vi "Main.vi"() -> ()   [LabVIEW 2025]
uses:
  Interlune UDP.ctl
  Enum_FileNewInterval.ctl
  <vilib>/DAQmx/read.llb/DAQmx Read (Analog 1D DBL NChan 1Samp).vi
  <vilib>/numeric/Random Number (Range) DBL.vi
  <extravilib>/ChannelInstances/Stream-a[.](dbl)/Read With Abort.vi
  <extravilib>/ChannelInstances/Stream-a[.](dbl)/Write With Abort.vi
  <extravilib>/ChannelInstances/Stream-a[.](dbl)/EndpointRead.vi
  <extravilib>/ChannelInstances/Stream-a[.](dbl)/Endpoint.vi
  <vilib>/DAQmx/miscellaneous.llb/DAQmx Fill In Error Info.vi
  <extravilib>/ChannelInstances/Stream-a[.](dbl)/Instantiate.vi
  <extravilib>/ChannelInstances/Stream-a[.](dbl)/)Channel.vi
  <resource>/ChannelSupport/_ChannelSupport/WaitIfNeeded.vi
  <extravilib>/ChannelInstances/Stream-a[.](dbl).lvlib
panel:
  in  "Output tabs":enum32{"Raw", "Cleaned"}(tab)
  out "LC Voltage Graph":T1(graph)
  out "Raw Voltages":dbl[](array[numeric])
  out "RAW UDP":string
  out "T Voltage Graph":cluster{"[0]":dbl}(graph)
  out "UDP Cluster":T2
  out "Forces":dbl[](array[numeric])
  out "LC Graph":T1(graph)
  out "T Graph":cluster{"[0]":dbl}(graph)
  in  "Load Cell Labeling":string[](array[string])=["LV1X", "LV1Y", "LV1Z", "LV2X", "LV2Y", "LV2Z", "LV3X", "LV3Y", "LV3Z", "LV4X", "LV4Y", "LV4Z"]
  in  "Torque Sensor":tag="cDAQ1Mod2/ai1"
  out "Time(s)":dbl
  in  "Emulation?":bool
  in  "Stop?":bool
  in  "Load Cells":tag[](array[tag])=["cDAQ1Mod1/ai5", "cDAQ1Mod1/ai4", "cDAQ1Mod1/ai6", "cDAQ1Mod1/ai8", "cDAQ1Mod1/ai7", "cDAQ1Mod1/ai9", "cDAQ1Mod1/ai11", "cDAQ1Mod1/ai10", "cDAQ1Mod1/ai12", "cDAQ1Mod1/ai14", "cDAQ1Mod1/ai13", "cDAQ1Mod1/ai15"]
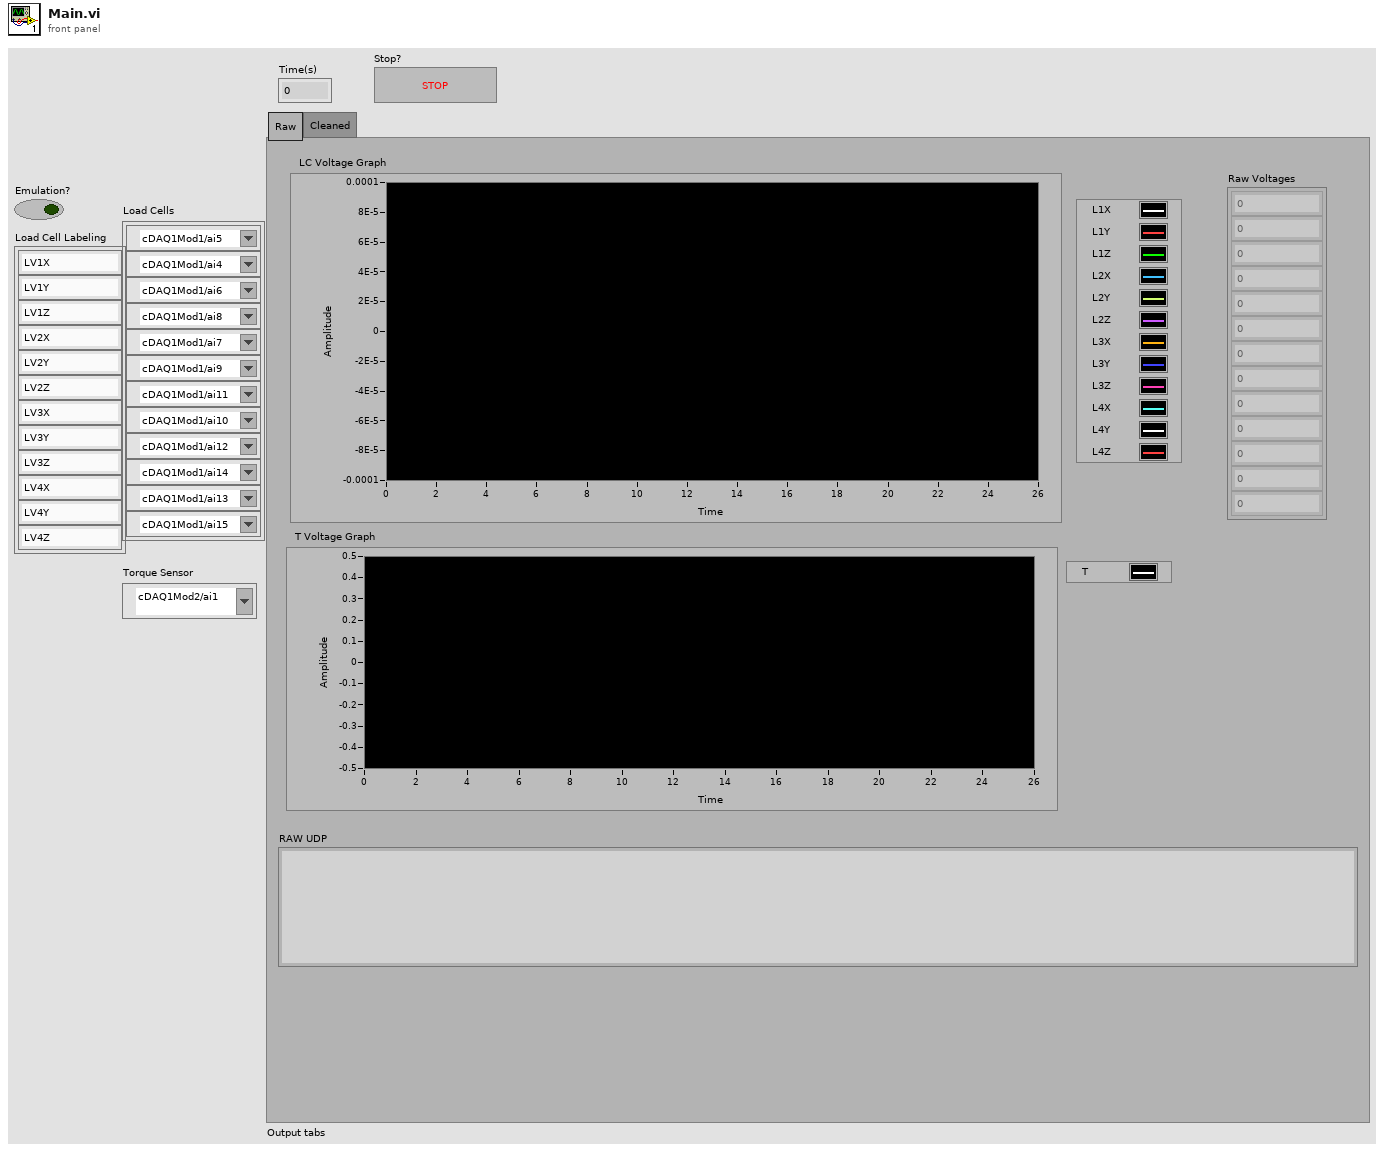
[diagram p1: front panel]
types:
  T1 = cluster{"[0]":dbl, "[1]":dbl, "[2]":dbl, "[3]":dbl, "[4]":dbl, "[5]":dbl, "[6]":dbl, "[7]":dbl, "[8]":dbl, "[9]":dbl, "[10]":dbl, "[11]":dbl}
  T2 = typedef "Interlune UDP.ctl" = cluster{"status":cluster{"ts_ms":dbl, "hw_estop":dbl, "motor_count":dbl}, "vertical":cluster{"has_v":dbl, "cmd":dbl, "raw_cmd":dbl, "velocity":dbl, "raw_velocity":dbl, "local_position":dbl, "global_position":dbl, "raw_position":dbl, "torque":dbl}, "horizontal":cluster{"has_h":dbl, "cmd":dbl, "raw_cmd":dbl, "velocity":dbl, "raw_velocity":dbl, "local_position":dbl, "global_position":dbl, "raw_position":dbl, "torque":dbl}, "attachment":cluster{"has_a":dbl, "cmd":dbl, "raw_cmd":dbl, "velocity":dbl, "raw_velocity":dbl, "global_position":dbl, "raw_position":dbl, "torque":dbl}}
  T3 = enum16{"open", "open or create", "create or replace", "create", "open (read-only)"}
  T4 = typedef "Enum_FileNewInterval.ctl" = enum16{"2 Min", "10 Min", "Hourly", "Daily", "Weekly", "Monthly"}
  T5 = typedef "Stream-a[.](dbl).lvlib/)Channel.ctl" = refnum<queue>
  T6 = cluster{"[0]":dbl, "[1]":dbl, "[2]":dbl, "[3]":dbl, "[4]":dbl, "[5]":dbl, "[6]":dbl, "[7]":dbl, "[8]":dbl, "[9]":dbl, "[10]":dbl, "[11]":dbl, "[12]":dbl}
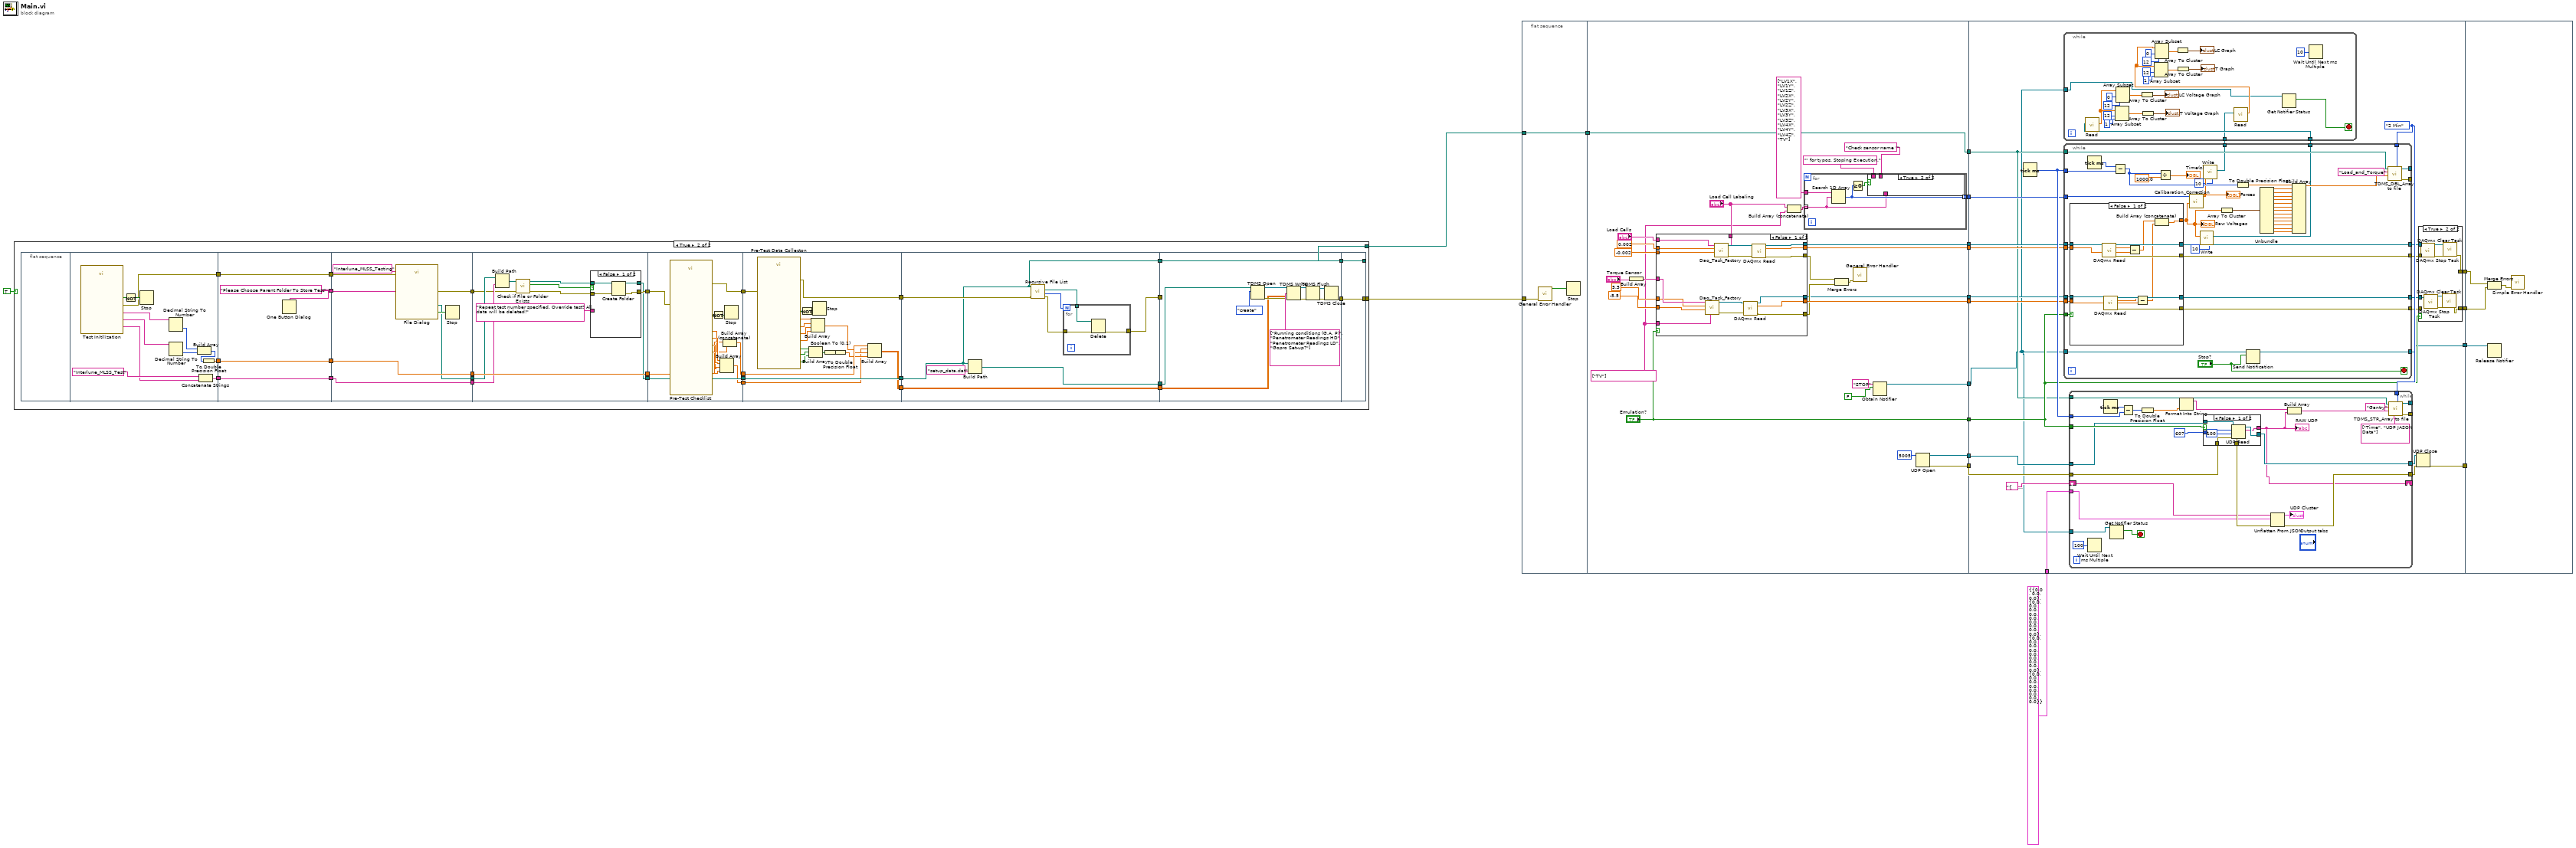
[diagram p0: block diagram]
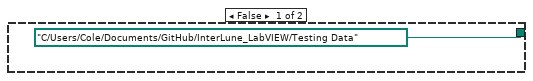
[diagram p2: hidden frame]
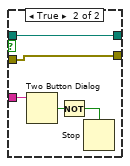
[diagram p3: hidden frame]
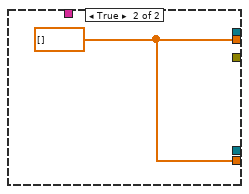
[diagram p4: hidden frame]
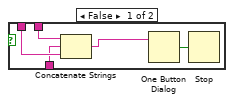
[diagram p5: hidden frame]
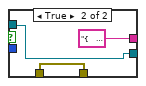
[diagram p7: hidden frame]
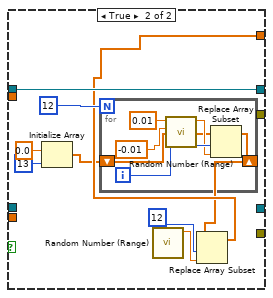
[diagram p8: hidden frame]
diagram:
  n1 = case shown="True" TRUE {
    tunnel: [_ w29] -> w12
    tunnel: [path "C:/Users/Cole/Documents/GitHub/InterLune_LabVIEW/Testing Data" ("dup path") w28] -> w7
    frame False {
    }
    frame True {
      n2 = flat-sequence {
        tunnel: [w59] -> w49
        tunnel: [w53] -> w48
        tunnel: [w50] -> w47
        tunnel: w49 -> [w64]
        tunnel: [w65] -> w46
        tunnel: [w64] -> w45
        tunnel: [w63] -> w44
        tunnel: w48 -> [w63]
        tunnel: [w62] -> w43
        tunnel: w47 -> [w62]
        tunnel: w46 -> [w73]
        tunnel: w45 -> [w72]
        tunnel: [w69] -> w42
        tunnel: [w68] -> w41
        tunnel: w44 -> [w68]
        tunnel: [w67] -> w40
        tunnel: w43 -> [w66]
        tunnel: [w66] -> w39
        tunnel: w42 -> [w80]
        tunnel: w41 -> [w84]
        tunnel: [w84] -> w27
        tunnel: w40 -> [w83]
        tunnel: [w74] -> w25
        tunnel: w39 -> [w82]
        tunnel: [w76] -> w23
        tunnel: w27 -> [w96]
        tunnel: [w94] -> w26
        tunnel: w25 -> [w106]
        tunnel: [w106] -> w24
        tunnel: w23 -> [w105]
        tunnel: [w104] -> w22
        tunnel: [w98] -> w21
        tunnel: w26 -> [w113]
        tunnel: w24 -> [w112]
        tunnel: [w112] -> w38
        tunnel: [w111] -> w37
        tunnel: [w110] -> w36
        tunnel: w22 -> [w114]
        tunnel: w21 -> [w107]
        tunnel: w38 -> [w126]
        tunnel: w37 -> [w129]
        tunnel: [w127] -> w35
        tunnel: w36 -> [w134]
        tunnel: [w134] -> w34
        tunnel: [w128] -> w33
        tunnel: [w126] -> w32
        tunnel: w35 -> [_]
        tunnel: w34 -> [w140]
        tunnel: w33 -> [w139]
        tunnel: [w141] -> w31
        tunnel: [w138] -> w30
        tunnel: w32 -> [w138]
        tunnel: [w151] -> w29
        tunnel: w31 -> [w151]
        tunnel: [w150] -> w28
        tunnel: w30 -> [w150]
        frame #0 {
        }
        frame #1 {
          n3 = call "Test Initilization"() -> ("Auger Speed"=w57:string, "Gantry Speed"=w58:string, "Test Number"=w51:string, "Done"=w60:bool, "error out"=w59:errorcluster)  [unwired: 15 in]
          n4 = Not(x=w60) -> (.not. x?=w61:bool)
          n5 = Stop(stop? (T)=w61) -> ()
          n6 = Decimal String To Number(string=w58) -> (number=w56:i32)  [unwired: 2 in, 1 out]
          n7 = Decimal String To Number(string=w57) -> (number=w55:i32)  [unwired: 2 in, 1 out]
          n8 = Build Array(w56, w55) -> (w54:i32[])
          n9 = Concatenate Strings("Interlune_MLSS_Test" ("default name"), w51) -> (w50:string)
          n10 = To Double Precision Float(number=w54) -> (double precision float=w53:dbl[])
        }
        frame #2 {
          w65 = "Please Choose Parent Folder To Store Test" ("prompt")
          n11 = One Button Dialog(message=w65) -> ()  [unwired: 1 in, 1 out]
        }
        frame #3 {
          n12 = call "File Dialog"("prompt"=w73, "default name"="Interlune_MLSS_Testing", "error in"=w72) -> ("selected path"=w67:path, "cancelled"=w71:bool, "error out"=w69:errorcluster)  [unwired: 9 in, 1 out]
          n13 = Stop(stop? (T)=w71) -> ()
        }
        frame #4 {
          n14 = Build Path(base path=w83, name or relative path=w82) -> (appended path=w81:path)
          n15 = call <vilib>:"Check if File or Folder Exists.vi"("error in (no error)"=w80, "path"=w81) -> ("error out"=w77:errorcluster, "file or folder exists?"=w75:bool, "dup path"=w78:path)  [unwired: 7 in]
          n16 = case shown="False" w75 {
            tunnel: [w88 w90] -> w74
            tunnel: "Repeat test number specified. Override test? All data will be deleted!" -> [_ w91]
            tunnel: [w87 w89] -> w76
            tunnel: w78 -> [w86 w90]
            tunnel: w77 -> [w85 w89]
            frame False {
              n17 = Create Folder(path (use dialog)=w86, error in=w85) -> (created path=w88:path, error out=w87:errorcluster)  [unwired: 1 in, 1 out]
            }
            frame True {
              n18 = Two Button Dialog(message=w91) -> (T button?=w92:bool)  [unwired: 2 in]
              n19 = Not(x=w92) -> (.not. x?=w93:bool)
              n20 = Stop(stop? (T)=w93) -> ()
            }
          }
        }
        frame #5 {
          n21 = call "Pre-Test Checklist"("error in (no error)"=w105) -> ("Penetrometer Reading in Track 4s"=w97:dbl, "Penetrometer Reading in Track 3"=w99:dbl, "Penetrometer Reading in Track 2"=w100:dbl, "Penetrometer Reading in Track 1"=w101:dbl, "Penetrometer Reading in Track Ref"=w95:dbl, "OK"=w102:bool, "error out"=w104:errorcluster)  [unwired: 8 in, 4 out]
          n22 = Not(x=w102) -> (.not. x?=w103:bool)
          n23 = Build Array(w101, w100, w99, w97) -> (w98:dbl[])
          n24 = Build Array (concatenate)(w96, w95) -> (w94:dbl[])
          n25 = Stop(stop? (T)=w103) -> ()
        }
        frame #6 {
          n26 = call "Pre-Test Data Collecton"("error in (no error)"=w114) -> ("Gantry Mounted Gopro"=w123:bool, "Hand-held Gopro"=w124:bool, "Wide FOV static Gopro"=w125:bool, "Penetromerter reading 4"=w116:dbl, "Penetrometer reading 3"=w117:dbl, "Penetrometer reading 2"=w118:dbl, "Penetrometer reading 1"=w119:dbl, "OK"=w121:bool, "error out"=w111:errorcluster)  [unwired: 10 in]
          n27 = Not(x=w121) -> (.not. x?=w120:bool)
          n28 = Build Array(w125, w124, w123) -> (w122:bool[])
          n29 = Build Array(w119, w118, w117, w116) -> (w109:dbl[])
          n30 = Stop(stop? (T)=w120) -> ()
          n31 = Boolean To (0,1)(Boolean=w122) -> (0, 1=w115:i16[])
          n32 = To Double Precision Float(number=w115) -> (double precision float=w108:dbl[])
          n33 = Build Array(w113, w107, w109, w108) -> (w110:dbl[][])
        }
        frame #7 {
          n34 = Build Path(base path=w126, name or relative path="setup_data.dat") -> (appended path=w128:path)
          n35 = call <vilib>:"Recursive File List.vi"("error in (no error)"=w129, "Folder Path"=w126) -> ("error out"=w130:errorcluster, "Number of Files"=w132:i32, "All Files in Dir"=w131:path[])  [unwired: 5 in, 2 out]
          n36 = for {
            N: w132 -> [_]
            tunnel: w131 -> [w137] mode=indexing
            tunnel: w130 -> [w136]
            tunnel: [w135] -> w127
            n37 = Delete(path (use dialog)=w137, error in=w136) -> (error out=w135:errorcluster)  [unwired: 3 in, 2 out]
          }
        }
        frame #8 {
          n38 = TDMS Open(10:T3."create" ("operation (0:open)"), 11:w139) -> (0:w142:errorcluster, 3:w145:refnum<k34>)  [unwired: 5 in]
          n39 = TDMS Write(0:w145, 7:string[] ["Running conditions (G,A, P)", "Penetrometer Readings HD", "Penetrometer Readings LD", "Gopro Set-up?"] ("channel name(s) in (Untitled)"), 9:w140, 11:w142) -> (4:w147:refnum<k34>, 15:w146:errorcluster)  [unwired: 2 in, 2 out]
          n40 = TDMS Flush(4:w146, 7:w147) -> (0:w148:errorcluster, 3:w149:refnum<k34>)
          n41 = TDMS Close(8:w148, 11:w149) -> (0:w141:errorcluster)  [unwired: 1 out]
        }
        frame #9 {
        }
      }
    }
  }
  n42 = flat-sequence {
    tunnel: w12 -> [w154]
    tunnel: w7 -> [w152]
    tunnel: [w152] -> w8
    tunnel: [w182] -> w19
    tunnel: [w181] -> w18
    tunnel: [w173] -> w17
    tunnel: [w171] -> w16
    tunnel: [w172] -> w15
    tunnel: ["Emulation?"] -> w14
    tunnel: [w169] -> w13
    tunnel: [w165] -> w9
    tunnel: w8 -> [w165]
    tunnel: [w161] -> w4
    tunnel: [w155] -> w2
    tunnel: w19 -> [w235]
    tunnel: w18 -> [w234]
    tunnel: w17 -> [w233]
    tunnel: w16 -> [w229]
    tunnel: w15 -> [w230]
    tunnel: w14 -> [w226]
    tunnel: w13 -> [w224]
    tunnel: [w228] -> w11
    tunnel: [w227] -> w10
    tunnel: w9 -> [w223]
    tunnel: T2 {"status"={"ts_ms"=0.0, "hw_estop"=0.0, "motor_count"=0.0}, "vertical"={"has_v"=0.0, "cmd"=0.0, "raw_cmd"=0.0, "velocity"=0.0, "raw_velocity"=0.0, "local_position"=0.0, "global_position"=0.0, "raw_position"=0.0, "torque"=0.0}, "horizontal"={"has_h"=0.0, "cmd"=0.0, "raw_cmd"=0.0, "velocity"=0.0, "raw_velocity"=0.0, "local_position"=0.0, "global_position"=0.0, "raw_position"=0.0, "torque"=0.0}, "attachment"={"has_a"=0.0, "cmd"=0.0, "raw_cmd"=0.0, "velocity"=0.0, "raw_velocity"=0.0, "global_position"=0.0, "raw_position"=0.0, "torque"=0.0}} ("Cluster") -> [w217]
    tunnel: w4 -> [w221]
    tunnel: [w218] -> w3
    tunnel: w2 -> [w215]
    tunnel: [w214] -> w1
    tunnel: w11 -> [w386]
    tunnel: w10 -> [_]
    tunnel: w3 -> [w385]
    tunnel: w1 -> [w383]
    frame #0 {
      n43 = call <vilib>:"General Error Handler.vi"("error in (no error)"=w154) -> ("error?"=w153:bool)  [unwired: 10 in, 4 out]
      n44 = Stop(stop? (T)=w153) -> ()
    }
    frame #1 {
      w158 = string[] ["TV"] ("Channel Names")
      n45 = Build Array("Torque Sensor") -> (w174:tag[])
      n46 = case shown="False" "Emulation?" {
        tunnel: "Load Cells" -> [w199 _]
        tunnel: 0.002 ("maximum value") -> [w198 _]
        tunnel: -0.002 ("minimum value") -> [w197 _]
        tunnel: 5.5 ("maximum value") -> [w186 _]
        tunnel: -5.5 ("minimum value") -> [w185 _]
        tunnel: w174 -> [w187 _]
        tunnel: [w196 _] -> w173
        tunnel: [w195 _] -> w164
        tunnel: "Load Cell Labeling" -> [w194 _]
        tunnel: [w193 w202] -> w172
        tunnel: [w190 w202] -> w171
        tunnel: w158 -> [w184 _]
        tunnel: [w189 _] -> w161
        tunnel: [w188 _] -> w162
        frame False {
          n47 = call "Daq_Task_Factory.vi"("Channel Names"=w184, "minimum value"=w185, "maximum value"=w186, "DAQmx Physical Channels"=w187) -> ("error out"=w191:errorcluster, "DAQmx Task Name"=w192:refnum<k21>)  [unwired: 6 in]
          n48 = call "Daq_Task_Factory.vi"("Channel Names"=w194, "minimum value"=w197, "maximum value"=w198, "DAQmx Physical Channels"=w199) -> ("error out"=w200:errorcluster, "DAQmx Task Name"=w201:refnum<k21>)  [unwired: 6 in]
          n49 = call-poly <vilib>:"DAQmx Read.vi"("task/channels in"=w192, "error in"=w191) -> ("task out"=w189:refnum<k21>, "data"=w190:dbl[], "error out"=w188:errorcluster)  [unwired: 11 in]
          n50 = call-poly <vilib>:"DAQmx Read.vi"("task/channels in"=w201, "error in"=w200) -> ("task out"=w196:refnum<k21>, "data"=w193:dbl[], "error out"=w195:errorcluster)  [unwired: 11 in]
        }
        frame True {
          w202 = dbl[] [] ("data")
        }
      }
      n51 = Build Array (concatenate)("Load Cell Labeling", w158) -> (w160:string[])
      n52 = for {
        tunnel: w160 -> [w203] mode=indexing
        tunnel: string[] ["LV1X", "LV1Y", "LV1Z", "LV2X", "LV2Y", "LV2Z", "LV3X", "LV3Y", "LV3Z", "LV4X", "LV4Y", "LV4Z", "TV"] ("Load Cell Labeling") -> [w208]
        tunnel: [w207] -> w169 mode=indexing
        tunnel: "Check sensor name '" -> [w205]
        tunnel: "' for typos. Stoping Execution." -> [w204]
        n53 = Search 1D Array(1D array=w208, element=w203) -> (index of element=w207:i32)  [unwired: 1 in]
        n54 = Greater Or Equal To 0?(x=w207) -> (x >= 0?=w206:bool)
        n55 = case shown="True" w206 {
          tunnel: w205 -> [w212 _]
          tunnel: w204 -> [w211 _]
          tunnel: w203 -> [w210 _]
          frame False {
            n56 = Concatenate Strings(w212, w210, w211) -> (w209:string)
            n57 = One Button Dialog(message=w209) -> (true=w213:bool)  [unwired: 1 in]
            n58 = Stop(stop? (T)=w213) -> ()
          }
          frame True {
          }
        }
      }
      n59 = Merge Errors(w164, w162) -> (w163:errorcluster)
      n60 = call <vilib>:"General Error Handler.vi"("error in (no error)"=w163) -> ()  [unwired: 10 in, 5 out]
      n61 = Obtain Notifier(name (unnamed)="STOP", notification data type=FALSE ("Emulation?")) -> (notifier out=w155:refnum<notifier>)  [unwired: 2 in, 2 out]
      n62 = UDP Open(11:u16 5005 ("port")) -> (port=w182:refnum<k16>, 0:w181:errorcluster)  [unwired: 4 in, 1 out]
    }
    frame #2 {
      w236 = Enum_FileNewInterval."2 Min" ("Interval")
      n63 = Tick Count (ms)() -> (millisecond timer value=w237:u32)
      n64 = while {
        tunnel: [w354] -> _
        tunnel: [w353] -> _
        tunnel: w237 -> [w351]
        tunnel: w236 -> [w343]
        tunnel: w226 -> [w342]
        tunnel: w233 -> [w330]
        tunnel: w229 -> [w326]
        tunnel: w230 -> [w327]
        tunnel: [w329] -> w231
        tunnel: [w328] -> w232
        tunnel: w224 -> [w325]
        tunnel: w223 -> [w323]
        tunnel: [w321] -> w225
        tunnel: [w318] -> w222
        tunnel: w221 -> [w315]
        tunnel: [w314] -> w220
        tunnel: [w313] -> w219
        tunnel: w215 -> [w312]
        tunnel: [w310] -> w214
        stop <- "Stop?" stop-if-true
        n65 = case shown="False" w342 {
          tunnel: [w356 w372] -> w319
          tunnel: w330 -> [w367 w376]
          tunnel: [w366 w376] -> w329
          tunnel: [w365 _] -> w328
          tunnel: w327 -> [w363 _]
          tunnel: w326 -> [w359 _]
          tunnel: w315 -> [w362 _]
          tunnel: [w361 _] -> w314
          tunnel: [w360 _] -> w313
          frame False {
            n66 = call-poly <vilib>:"DAQmx Read.vi"("task/channels in"=w367) -> ("task out"=w366:refnum<k21>, "data"=w364:dbl[], "error out"=w365:errorcluster)  [unwired: 12 in]
            n67 = call-poly <vilib>:"DAQmx Read.vi"("task/channels in"=w362) -> ("task out"=w361:refnum<k21>, "data"=w358:dbl[], "error out"=w360:errorcluster)  [unwired: 12 in]
            n68 = Subtract(x=w364, y=w363) -> (x-y=w357:dbl[])
            n69 = Subtract(x=w358, y=w359) -> (x-y=w355:dbl[])
            n70 = Build Array (concatenate)(w357, w355) -> (w356:dbl[])
          }
          frame True {
            n71 = Initialize Array(0.0 ("element"), 13 ("dimension size")) -> (w370:dbl[])
            n72 = for {
              N: 12 -> [_]
              shift-right: [w377] -> w371
              shift-left: w370 -> [w378]
              i -> [w380]
              n73 = call-poly <vilib>:"Random Number (Range).vi"("lower bound (0)"=-0.01 ("upper bound (100)"), "upper bound (100)"=0.01) -> ("number"=w379:dbl)  [unwired: 9 in]
              n74 = Replace Array Subset(array=w378, new element=w379, index=w380) -> (w377:dbl[])
            }
            n75 = call-poly <vilib>:"Random Number (Range).vi"() -> ("number"=w374:dbl)  [unwired: 11 in]
            n76 = Replace Array Subset(array=w371, new element=w374, index=12) -> (w372:dbl[])
          }
        }
        "Raw Voltages" <- w319
        n77 = Tick Count (ms)() -> (millisecond timer value=w352:u32)
        n78 = Subtract(x=w352, y=w351) -> (x-y=w332:u32)
        n79 = Divide(x=w332, y=1000.0) -> (x/y=→"Time(s)":dbl)
        n80 = call "Calibaration_Correction.vi"("data"=w319, "Index Map"=w325) -> ("Calibrated Array"=w320:dbl[])  [unwired: 9 in]
        "Forces" <- w320
        n81 = call <extravilib>:"Write.vi"("size (unlimited)"=10, "element"=w319) -> ("channel"=w321:T5)  [unwired: 7 in, 2 out]
        n82 = call <extravilib>:"Write.vi"("size (unlimited)"=10, "element"=w320) -> ("channel"=w318:T5)  [unwired: 7 in, 2 out]
        n83 = Array To Cluster(array=w319) -> (cluster=w322:T6)
        n84 = To Double Precision Float(number=w332) -> (double precision float=w349:dbl)
        n85 = Send Notification(notification="Stop?", notifier=w312) -> (notifier out=w310:refnum<notifier>)  [unwired: 1 in, 1 out]
        n86 = Unbundle(w322) -> ("[0]"=w348:dbl, "[1]"=w347:dbl, "[2]"=w346:dbl, "[3]"=w345:dbl, "[4]"=w344:dbl, "[5]"=w341:dbl, "[6]"=w340:dbl, "[7]"=w339:dbl, "[8]"=w338:dbl, "[9]"=w337:dbl, "[10]"=w336:dbl, "[11]"=w335:dbl, "[12]"=w334:dbl)
        n87 = Build Array(w349, w348, w347, w346, w345, w344, w341, w340, w339, w338, w337, w336, w335, w334) -> (w350:dbl[])
        n88 = call "TDMS_DBL_Array to file.vi"("Interval"=w343, "Data"=w350, "FilePrefix"="Load_and_Torque", "Base path"=w323) -> ("error out"=w353:errorcluster, "sonic file out"=w354:refnum<k34>)  [unwired: 6 in]
      }
      n89 = while {
        tunnel: w225 -> [w258]
        tunnel: w222 -> [w244]
        tunnel: w215 -> [w241]
        stop <- w240 stop-if-true
        n90 = call <extravilib>:"Read.vi"("channel"=w258) -> ("element"=w254:dbl[])  [unwired: 6 in, 4 out]
        n91 = Array Subset(array=w254, index=12, length=1) -> (w253:dbl[])
        n92 = Array Subset(array=w254, index=0, length=12) -> (w252:dbl[])
        n93 = Array To Cluster(array=w252) -> (cluster=→"LC Voltage Graph":T1)
        n94 = Array To Cluster(array=w253) -> (cluster=→"T Voltage Graph":cluster{"[0]":dbl})
        n95 = call <extravilib>:"Read.vi"("channel"=w244) -> ("element"=w243:dbl[])  [unwired: 6 in, 4 out]
        n96 = Array Subset(array=w243, index=12, length=1) -> (w246:dbl[])
        n97 = Array Subset(array=w243, index=0, length=12) -> (w247:dbl[])
        n98 = Array To Cluster(array=w247) -> (cluster=→"LC Graph":T1)
        n99 = Array To Cluster(array=w246) -> (cluster=→"T Graph":cluster{"[0]":dbl})
        n100 = Get Notifier Status(notifier=w241) -> (current notification=w240:bool)  [unwired: 1 in, 4 out]
        n101 = Wait Until Next ms Multiple(millisecond multiple=u32 10) -> ()  [unwired: 1 out]
      }
      n102 = while {
        tunnel: [w296] -> _
        tunnel: [w295] -> _
        tunnel: w236 -> [w293]
        tunnel: w237 -> [w298]
        tunnel: w226 -> [w289]
        tunnel: w235 -> [w286]
        tunnel: w234 -> [w288]
        tunnel: [w285] -> w238
        tunnel: [w281] -> w239
        tunnel: w223 -> [w280]
        tunnel: w217 -> [w279]
        shift-right: [w278] -> _
        shift-left: "{    \"status\": {        \"ts_ms\": -1,        \"hw_estop\": -1,        \"motor_count\": -1    },    \"horizontal\": {        \"has_h\": -1,        \"cmd\": -1,        \"raw_cmd\": -1,        \"velocity\": -1,        \"raw_velocity\": -1,        \"raw_position\": -1,        \"global_position\": -1,        \"local_position\": -1,        \"torque\": -1    },    \"vertical\": {        \"has_v\": -1,        \"cmd\": -1,        \"raw_cmd\": -1,        \"velocity\": -1,        \"raw_velocity\": -1,        \"raw_position\": -1,        \"global_position\": -1,        \"local_position\": -1,        \"torque\": -1    },    \"attachment\": {        \"has_a\": -1,        \"cmd\": -1,        \"raw_cmd\": -1,        \"velocity\": -1,        \"raw_velocity\": -1,        \"raw_position\": -1,        \"global_position\": -1,        \"torque\": -1    }}" -> [w277]
        tunnel: w215 -> [w276]
        stop <- w275 stop-if-true
        n103 = Wait Until Next ms Multiple(millisecond multiple=u32 100) -> ()  [unwired: 1 out]
        n104 = Tick Count (ms)() -> (millisecond timer value=w299:u32)
        n105 = Get Notifier Status(notifier=w276) -> (current notification=w275:bool)  [unwired: 1 in, 4 out]
        n106 = Subtract(x=w299, y=w298) -> (x-y=w297:u32)
        n107 = To Double Precision Float(number=w297) -> (double precision float=w291:dbl)
        n108 = Format Into String(w291) -> (resulting string=w290:string)  [unwired: 3 in, 1 out]
        n109 = case shown="False" w289 {
          tunnel: [w301 "{    \"status\": {        \"ts_ms\": -1,        \"hw_estop\": -1,        \"motor_count\": -1    },    \"horizontal\": {        \"has_h\": -1,        \"cmd\": -1,        \"raw_cmd\": -1,        \"velocity\": -1,        \"raw_velocity\": -1,        \"raw_position\": -1,        \"global_position\": -1,        \"local_position\": -1,        \"torque\": -1    },    \"vertical\": {        \"has_v\": -1,        \"cmd\": -1,        \"raw_cmd\": -1,        \"velocity\": -1,        \"raw_velocity\": -1,        \"raw_position\": -1,        \"global_position\": -1,        \"local_position\": -1,        \"torque\": -1    },    \"attachment\": {        \"has_a\": -1,        \"cmd\": -1,        \"raw_cmd\": -1,        \"velocity\": -1,        \"raw_velocity\": -1,        \"raw_position\": -1,        \"global_position\": -1,        \"torque\": -1    }}"] -> w278
          tunnel: w288 -> [w306 w309]
          tunnel: 607 ("max size (548)") -> [w305 _]
          tunnel: w286 -> [w304 w308]
          tunnel: [w303 w309] -> w282
          tunnel: [w302 w308] -> w285
          frame False {
            n110 = UDP Read(connection ID=w304, max size (548)=w305, timeout ms (25000)=100, 8:w306) -> (data out=w301:string, error out=w303:errorcluster, 3:w302:refnum<k16>)  [unwired: 2 out]
          }
          frame True {
          }
        }
        "RAW UDP" <- w278
        n111 = Unflatten From JSON(JSON string=w277, type and defaults=w279, error in (no error)=w282) -> (value=→"UDP Cluster":T2, error out=w281:errorcluster)  [unwired: 4 in]
        n112 = Build Array(w290, w278) -> (w292:string[])
        n113 = call "TDMS_STR_Array to file.vi"("Interval"=w293, "channel name(s) in"=string[] ["Time", "UDP JASON Data"], "Data"=w292, "FilePrefix"="Gantry", "Base path"=w280) -> ("error out"=w295:errorcluster, "sonic file out"=w296:refnum<k34>)  [unwired: 5 in]
      }
      n114 = UDP Close(connection ID=w238, 8:w239) -> (error out=w227:errorcluster)  [unwired: 1 out]
      n115 = case shown="True" w226 {
        tunnel: w232 -> [w264 w271]
        tunnel: w231 -> [_ w270]
        tunnel: [w264 w269] -> w228
        tunnel: w220 -> [_ w266]
        tunnel: w219 -> [w263 _]
        tunnel: [w263 w265] -> w218
        frame False {
        }
        frame True {
          n116 = call <vilib>:"DAQmx Stop Task.vi"("task/channels in"=w270, "error in"=w271) -> ("task out"=w273:refnum<k21>, "error out"=w272:errorcluster)  [unwired: 12 in]
          n117 = call <vilib>:"DAQmx Stop Task.vi"("task/channels in"=w266) -> ("task out"=w267:refnum<k21>, "error out"=w268:errorcluster)  [unwired: 13 in]
          n118 = call <vilib>:"DAQmx Clear Task.vi"("task in"=w267, "error in"=w268) -> ("error out"=w265:errorcluster)  [unwired: 13 in]
          n119 = call <vilib>:"DAQmx Clear Task.vi"("task in"=w273, "error in"=w272) -> ("error out"=w269:errorcluster)  [unwired: 13 in]
        }
      }
    }
    frame #3 {
      n120 = Merge Errors(w386, w385) -> (w384:errorcluster)
      n121 = Release Notifier(notifier=w383) -> ()  [unwired: 2 in, 3 out]
      n122 = call <vilib>:"Simple Error Handler.vi"("error in (no error)"=w384) -> ()  [unwired: 4 in, 5 out]
    }
  }
